vi "End Log File.vi"(10 "Seconds":dbl, 11 "Muestras totales":i32) -> (3 "String":string)   [LabVIEW 2014]
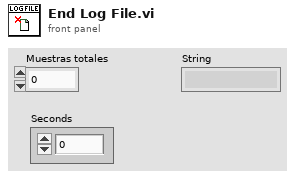
[diagram p1: front panel]
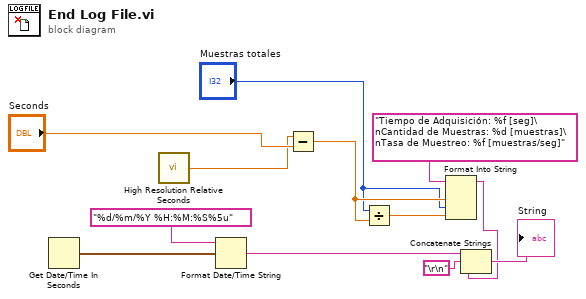
[diagram p0: block diagram]
diagram:
  n1 = Get Date/Time In Seconds() -> (seconds since 1Jan1904=w6:timestamp)
  n2 = call <vilib>:"High Resolution Relative Seconds.vi"() -> ("relative seconds"=w1:dbl)
  n3 = Format Date/Time String(time format string (%c)="%d/%m/%Y %H:%M:%S%5u" ("string"), seconds (now)=w6) -> (date/time string=w3:string)  [unwired: 1 in]
  n4 = Subtract(x=w1, y="Seconds") -> (x-y=w9:dbl)
  n5 = Divide(x="Muestras totales", y=w9) -> (x/y=w8:dbl)
  n6 = Format Into String(format string="Tiempo de Adquisición: %f [seg]\nCantidad de Muestras: %d [muestras]\nTasa de Muestreo: %f [muestras/seg]" ("string"), w9, "Muestras totales", w8) -> (resulting string=w11:string)  [unwired: 2 in, 1 out]
  n7 = Concatenate Strings(w3, "\r\n", w11) -> (→"String":string)
